vi "Read dta File.vi"(8 "错误输入":errorcluster, 11 "Path":path=path "E:/LCU6331 test/Procedure2/RFID_m645_Prodtest_LCU6331.128") -> (0 "错误输出":errorcluster, 1 "line size":i32, 2 "输出数组":string[](array[string]), 3 "path":path)   [LabVIEW 2009]
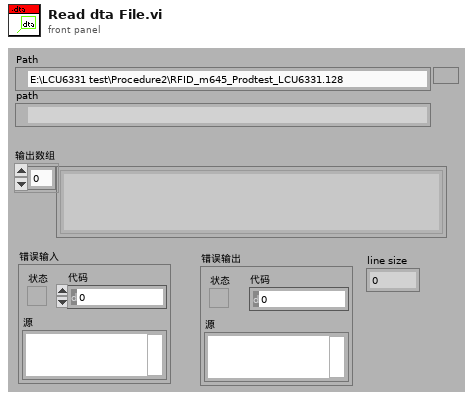
[diagram p1: front panel]
types:
  T1 = enum16{"open", "replace", "create", "open or create", "replace or create", "replace or create with confirmation"}
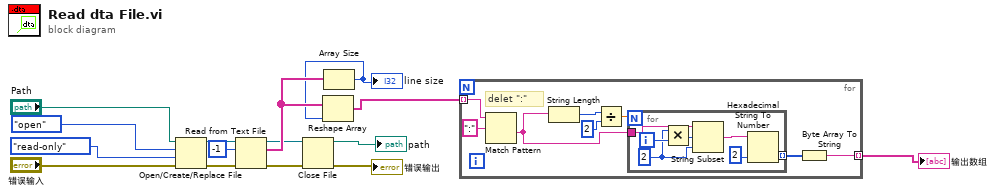
[diagram p0: block diagram]
diagram:
  n1 = Open/Create/Replace File(file path (use dialog)="Path", error in="错误输入", operation (0:open)=T1."open" ("操作(0:open)"), access (0:read/write)=enum16{"read/write", "read-only", "write-only"}."read-only" ("权限(0:read/write)")) -> (refnum out=w11:refnum<file>, error out=w12:errorcluster)  [unwired: 3 out]
  n2 = Read from Text File(file (use dialog)=w11, count=-1 ("计数"), error in=w12) -> (refnum out=w8:refnum<file>, text=w10:string[], error out=w7:errorcluster)  [unwired: 2 out]
  n3 = Close File(refnum=w8, error in=w7) -> (path=→"path":path, error out=→"错误输出":errorcluster)
  n4 = Array Size(array=w10) -> (size(s)=w5:i32)
  "line size" <- w5
  n5 = Reshape Array(w10, w5) -> (w2:string[])
  n6 = for {
    tunnel: w2 -> [w17] mode=indexing
    tunnel: [w19] -> w1 mode=indexing
    # "delet \":\""
    n7 = Match Pattern(string=w17, regular expression=":" ("search string/char (-)")) -> (after substring=w16:string)  [unwired: 4 out]
    n8 = String Length(string=w16) -> (length=w23:i32)
    n9 = Divide(x=w23, y=2) -> (x/y=w21:dbl)
    n10 = for {
      N: w21 -> [_]
      tunnel: w16 -> [w30]
      tunnel: [w25] -> w20 mode=indexing
      i -> [w29]
      w28 = 2 ("length (rest)")
      n11 = Multiply(x=w28, y=w29) -> (x*y=w27:i32)
      n12 = String Subset(string=w30, offset (0)=w27, length (rest)=w28) -> (substring=w26:string)
      n13 = Hexadecimal String To Number(string=w26, default (0uL)=u8 2) -> (number=w25:u8)  [unwired: 2 out]
    }
    n14 = Byte Array To String(unsigned byte array=w20) -> (string=w19:string)
  }
  "输出数组" <- w1
